vi "expanded sql.vi"(8 "error in (no error)":errorcluster, 11 "pStmt":dbl) -> (0 "error out":errorcluster, 2 "function return":string, 3 "pStmt out":dbl)   [LabVIEW 2020, in "sqlite3.lvlib"]
uses:
  sqlite3.lvlib
  errstr.vi
  bin/sqlite3_64.dll
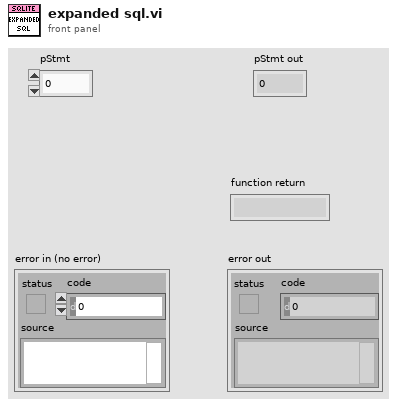
[diagram p1: front panel]
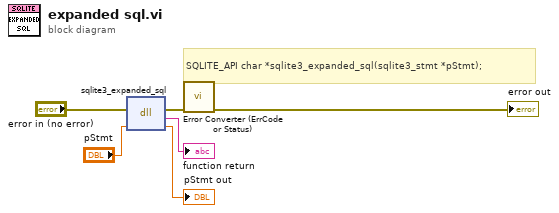
[diagram p0: block diagram]
diagram:
  # "SQLITE_API char *sqlite3_expanded_sql(sqlite3_stmt *pStmt);"
  n1 = dll-call lib="C:/Users/Fred.Guo/Desktop/Database-configuration/externals/sqlite3/Source/bin/sqlite3_*.*" fn="sqlite3_expanded_sql"(error in="error in (no error)", "pStmt"="pStmt") -> (error out=w2:errorcluster, →"function return":string, "pStmt"=→"pStmt out":dbl)  [unwired: 2 in, 1 out]
  n2 = call "Error Converter (ErrCode or Status).vi"("error in (no error)"=w2) -> ("error out"=→"error out":errorcluster)  [unwired: 10 in]
